vi "First.vi"(8 "Error In":errorcluster, 10 "Known Host In":refnum<class "Known Host.lvclass">, 11 "KnownHosts In":refnum<class "Known Hosts.lvclass">) -> (0 "Error Out":errorcluster, 1 "Result":T1, 2 "Known Host Out":refnum<class "Known Host.lvclass">, 3 "KnownHosts Out":refnum<class "Known Hosts.lvclass">)   [LabVIEW 2018, in "Toolkit.lvlib" / "Known Hosts.lvclass"]
uses:
  Known Hosts.lvclass
  Known Host/Known Host.lvclass
  Typedefs/Get Results.ctl
  Known Hosts.lvclass/Known Hosts.ctl
  Known Host/Known Host.lvclass/Known Host.ctl
  Session/Session.lvclass/Session.ctl
  SSH/SSH.lvclass/SSH.ctl
  Toolkit.lvlib
  Session/Session.lvclass
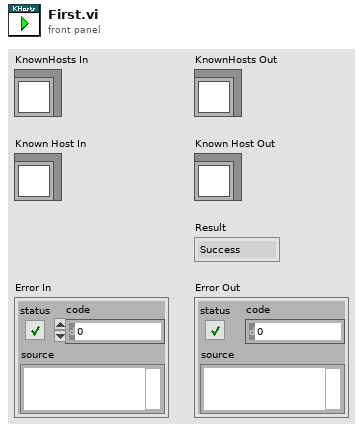
[diagram p1: front panel]
types:
  T1 = typedef "Toolkit.lvlib/Known Hosts.lvclass/Get Results.ctl" = enum32{"Success", "End of Hosts"}
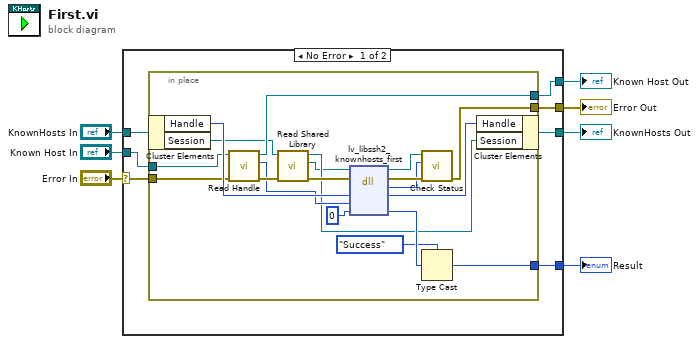
[diagram p0: block diagram]
diagram:
  n1 = case shown="No Error" "Error In" {
    selector: "Error In" -> [w12 w36]
    tunnel: "KnownHosts In" -> [w14 w35]
    tunnel: [w11 w36] -> w5
    tunnel: [w13 w35] -> w4
    tunnel: "Known Host In" -> [w10 w34]
    tunnel: [w9 w34] -> w2
    tunnel: [w8 _] -> w1
    frame No Error {
      n2 = in-place {
        in-place-border: w12 -> [w26]
        in-place-border: [w29] -> w11
        in-place-border: w10 -> [w27]
        in-place-border: [w23] -> w9
        in-place-border: [w19] -> w8
        n3 = in-place-cluster #1(w14) -> ("Handle"=w33:u64, "Session"=w17:refnum<class "Session.lvclass">)
        n4 = call "Read Handle.vi"("Error In"=w26, "Known Host In"=w27) -> ("Error Out"=w25:errorcluster, "Handle"=w24:u64, "Known Host Out"=w23:refnum<class "Known Host.lvclass">)  [unwired: 7 in]
        n5 = call "Read Shared Library.vi"("Error In"=w25, "Session In"=w17) -> ("Erorr Out"=w18:errorcluster, "libssh2lv Shared Library"=w15:path, "Session Out"=w16:refnum<class "Session.lvclass">)  [unwired: 7 in]
        n6 = dll-call lib="lv-libssh2.*" fn="lv_libssh2_knownhosts_first"(path in=w15, error in=w18, "handle"=w33, "host"=w24, "result"=0) -> (path out=w30:path, error out=w31:errorcluster, "status"=w28:i32, "handle"=w32:u64, "result"=w21:i32)  [unwired: 2 in]
        n7 = call "Check Status.vi"("Error In"=w31, "Status"=w28, "lv-libssh2 Shared Library In"=w30) -> ("Error Out"=w29:errorcluster)  [unwired: 7 in, 1 out]
        n8 = Type Cast(type=Get_Results."Success" ("Get Result"), x=w21) -> (*(type *) &x=w19:T1)
        n9 = in-place-cluster #1("Handle"=w32, "Session"=w16) -> (w13:refnum<class "Known Hosts.lvclass">)
      }
    }
    frame Error {
    }
  }
  "Error Out" <- w5
  "KnownHosts Out" <- w4
  "Known Host Out" <- w2
  "Result" <- w1
